vi "Finish.vi"(8 "error in (no error)":errorcluster, 11 "FileConfig in":refnum<class "FileConfig.lvclass">) -> (0 "error out":errorcluster, 3 "FileConfig out":refnum<class "FileConfig.lvclass">)   [LabVIEW 2018, in "Config.lvlib" / "FileConfig.lvclass"]
uses:
  FileConfig.lvclass
  FileConfig.lvclass/FileConfig.ctl
  Config.lvclass
  <vilib>/Utility/config.llb/NI_LVConfig.lvlib
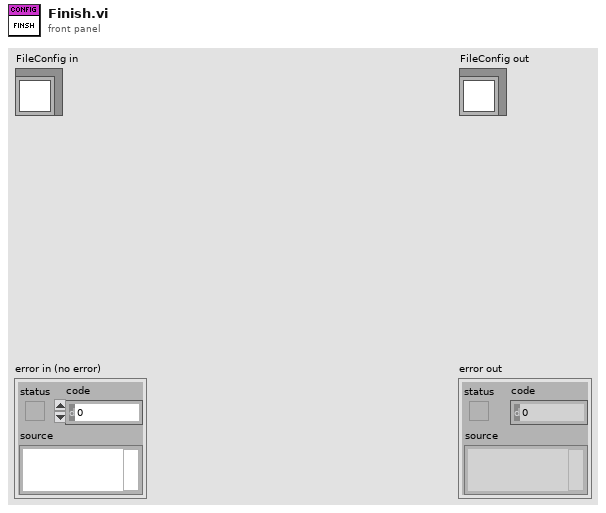
[diagram p1: front panel]
types:
  T1 = typedef "NI_LVConfig.lvlib/Config Data RefNum.ctl" = refnum<k1>
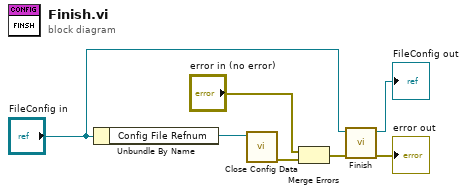
[diagram p0: block diagram]
diagram:
  n1 = Unbundle By Name("FileConfig in") -> ("Config File Refnum"=w3:T1)
  n2 = call <vilib>:"Close Config Data.vi"("refnum"=w3) -> ("error out"=w6:errorcluster)  [unwired: 9 in, 1 out]
  n3 = Merge Errors("error in (no error)", w6) -> (w2:errorcluster)
  n4 = call-parent "Finish.vi"("error in (no error)"=w2, "Config in"="FileConfig in") -> ("error out"=→"error out":errorcluster, "Config out"=→"FileConfig out":refnum<class "FileConfig.lvclass">)  [unwired: 8 in]
